vi "Test Circular Buffer.vi"() -> ()   [LabVIEW 2013]
uses:
  ByteFIFO/ByteFIFO.lvclass
  VariantBufferMap/VariantBufferMap.lvclass
  VariantBuffer/VariantBuffer.lvclass
  ObjectBuffer/ObjectBuffer.lvclass
panel:
  out "error Buffer already exists":errorcluster
  out "error MAP FULL":errorcluster
  out "Names":string[](array[string])
  out "element":variant
  out "data":string[](array[string])
  out "bytes":u8[](array[numeric]) format="%02x"
  in  "stop":bool
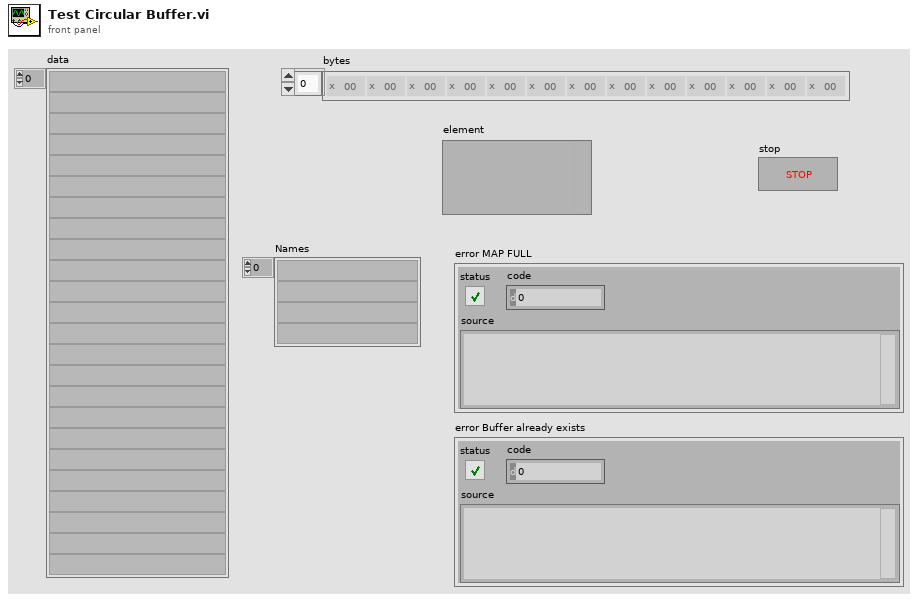
[diagram p1: front panel]
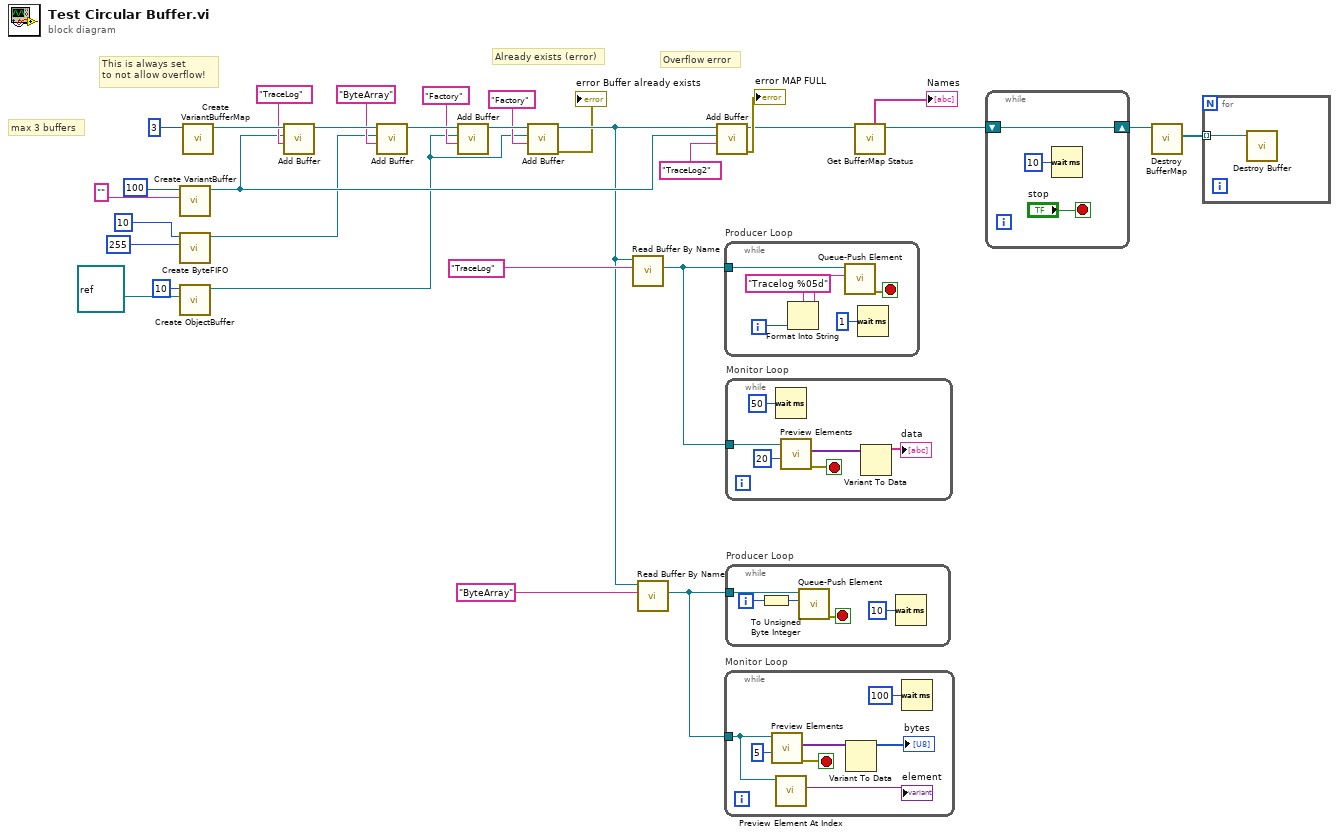
[diagram p0: block diagram]
diagram:
  # "Already exists (error)"
  # "Overflow error"
  # "This is always set\nto not allow overflow!"
  # "max 3 buffers"
  n1 = call "Create VariantBuffer.vi"("default"="", "bufSize"=100) -> ("Buffer"=w18:refnum<data-value>)  [unwired: 8 in, 1 out]
  n2 = call "Create ByteFIFO.vi"("default value"=u8 255, "bufSize"=10) -> ("Buffer"=w7:refnum<data-value>)  [unwired: 8 in, 1 out]
  n3 = call "Create ObjectBuffer.vi"("default"=refnum<class> refnum ("LabVIEW Object"), "bufSize"=10) -> ("Buffer"=w2:refnum<data-value>)  [unwired: 8 in, 1 out]
  n4 = call "Create VariantBufferMap.vi"("bufSize"=3) -> ("BufferMap"=w26:refnum<data-value>)  [unwired: 9 in, 1 out]
  n5 = call "Add Buffer.vi"("Name"="TraceLog", "Buffer"=w18, "BufferMap in"=w26) -> ("BufferMap"=w24:refnum<data-value>)  [unwired: 7 in, 1 out]
  n6 = call "Add Buffer.vi"("Name"="ByteArray", "Buffer"=w7, "BufferMap in"=w24) -> ("BufferMap"=w12:refnum<data-value>)  [unwired: 7 in, 1 out]
  n7 = call "Add Buffer.vi"("Name"="Factory", "Buffer"=w2, "BufferMap in"=w12) -> ("BufferMap"=w5:refnum<data-value>)  [unwired: 7 in, 1 out]
  n8 = call "Add Buffer.vi"("Name"="Factory", "Buffer"=w2, "BufferMap in"=w5) -> ("error out"=→"error Buffer already exists":errorcluster, "BufferMap"=w4:refnum<data-value>)  [unwired: 7 in]
  n9 = call "Read Buffer By Name.vi"("Name"="TraceLog", "BufferMap in"=w4) -> ("Buffer"=w9:refnum<data-value>)  [unwired: 6 in, 3 out]
  n10 = call "Read Buffer By Name.vi"("Name"="ByteArray", "BufferMap in"=w4) -> ("Buffer"=w6:refnum<data-value>)  [unwired: 6 in, 3 out]
  n11 = call "Add Buffer.vi"("Name"="TraceLog2", "Buffer"=w18, "BufferMap in"=w4) -> ("error out"=→"error MAP FULL":errorcluster, "BufferMap"=w15:refnum<data-value>)  [unwired: 7 in]
  n12 = while "Producer Loop" {
    tunnel: w9 -> [w34]
    i -> [w36]
    stop <- w32 stop-if-true
    n13 = Format Into String(format string="Tracelog %05d", w36) -> (resulting string=w33:string)  [unwired: 2 in, 1 out]
    n14 = call "Queue-Push Element.vi"("element"=w33, "Buffer in"=w34) -> ("error out"=w32:errorcluster)  [unwired: 6 in, 3 out]
    n15 = Wait (ms)(milliseconds to wait=u32 1) -> ()  [unwired: 1 out]
  }
  n16 = while "Monitor Loop" {
    tunnel: w6 -> [w42]
    stop <- w40 stop-if-true
    n17 = call "Preview Elements.vi"("count (-1: all)"=5, "ByteBuffer in"=w42) -> ("error out"=w40:errorcluster, "elements"=w39:variant[])  [unwired: 7 in, 1 out]
    n18 = call "Preview Element At Index.vi"("Buffer in"=w42) -> ("element"=→"element":variant)  [unwired: 7 in, 3 out]
    n19 = Variant To Data(Variant=w39) -> (data=→"bytes":u8[])  [unwired: 2 in, 1 out]
    n20 = Wait (ms)(milliseconds to wait=u32 100) -> ()  [unwired: 1 out]
  }
  n21 = while "Monitor Loop" {
    tunnel: w9 -> [w49]
    stop <- w48 stop-if-true
    n22 = Wait (ms)(milliseconds to wait=u32 50) -> ()  [unwired: 1 out]
    n23 = call "Preview Elements.vi"("count (-1: all)"=20, "ByteBuffer in"=w49) -> ("error out"=w48:errorcluster, "elements"=w46:variant[])  [unwired: 7 in, 1 out]
    n24 = Variant To Data(Variant=w46) -> (data=→"data":string[])  [unwired: 2 in, 1 out]
  }
  n25 = while "Producer Loop" {
    tunnel: w6 -> [w53]
    i -> [w54]
    stop <- w51 stop-if-true
    n26 = To Unsigned Byte Integer(number=w54) -> (unsigned 8bit integer=w52:u8)
    n27 = call "Queue-Push Element.vi"("element"=w52, "Buffer in"=w53) -> ("error out"=w51:errorcluster)  [unwired: 6 in, 3 out]
    n28 = Wait (ms)(milliseconds to wait=u32 10) -> ()  [unwired: 1 out]
  }
  n29 = call "Get BufferMap Status.vi"("BufferMap in"=w15) -> ("BufferMap"=w21:refnum<data-value>, "Names"=→"Names":string[])  [unwired: 5 in, 4 out]
  n30 = while {
    shift-right: [w56] -> w22
    shift-left: w21 -> [w56]
    stop <- "stop" stop-if-true
    n31 = Wait (ms)(milliseconds to wait=u32 10) -> ()  [unwired: 1 out]
  }
  n32 = call "Destroy BufferMap.vi"("Buffer"=w22) -> ("buffers"=w19:refnum<data-value>[])  [unwired: 8 in, 2 out]
  n33 = for {
    tunnel: w19 -> [w59] mode=indexing
    n34 = call "Destroy Buffer.vi"("Buffer"=w59) -> ()  [unwired: 9 in, 2 out]
  }
